vi "Constant_File Information Type.vi"() -> (0 "File Information Type":string[](array[string])=["Name", "Version", "Path"])   [LabVIEW 2015, in "File Version Lib.lvlib"]
uses:
  File Version Lib.lvlib
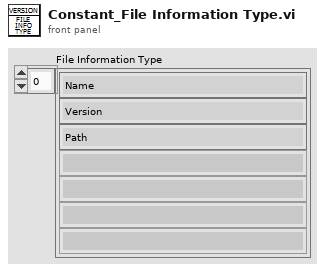
[diagram p1: front panel]
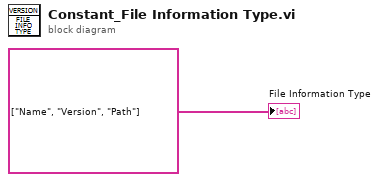
[diagram p0: block diagram]
diagram:
  "File Information Type" <- string[] ["Name", "Version", "Path"]
